vi "getFPGAReference.vi"(11 "TimestampControlFIFO in":refnum<class "TimestampControlFIFO.lvclass">) -> (2 "FPGAReference":refnum<k20>, 3 "TimestampControlFIFO out":refnum<class "TimestampControlFIFO.lvclass">)   [LabVIEW 2016]
uses:
  TimestampControlFIFO.lvclass
  D:/Code/ts_M1M3Support/Common_RT_FPGA/IWriteU64FIFO/IWriteU64FIFO.lvclass
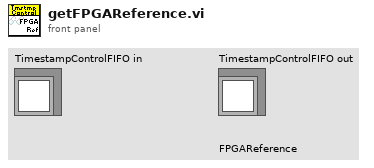
[diagram p1: front panel]
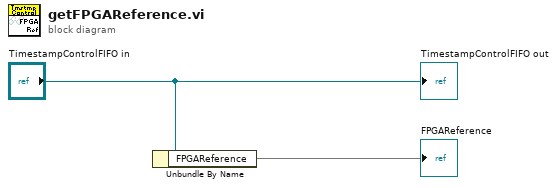
[diagram p0: block diagram]
diagram:
  n1 = Unbundle By Name("TimestampControlFIFO in") -> ("FPGAReference"=→"FPGAReference")
  "TimestampControlFIFO out" <- "TimestampControlFIFO in"
